vi "Calc_Remaining_Time.vi"(0 "Table In":T1[](array[typedef]) {"Carrier_2 Q (l/min)" format="%#.2f"; "Row Duration (mins)" format="%#.1f"; "Row No" min=0; "Trace Gas Concentration (%)" min=0.0 format="%#_4f"; "Carrier_1 Q (l/min)" format="%#.4f"; "Start X" format="%#.2f"; "Start Y" format="%#.2f"; "Start Z" format="%#.2f"; "End X" format="%#.2f"; "End Y" format="%#.2f"; "End Z" format="%#.2f"; "Tunnel Speed" format="%#.2f"; "Averaging time (mins)" min=0.0 format="%#.2f"}, 1 "Currently on Row":i32) -> (2 "Table Out":T1[](array[typedef]) {"Carrier_2 Q (l/min)" format="%#.2f"; "Row Duration (mins)" format="%#.1f"; "Row No" min=0; "Trace Gas Concentration (%)" min=0.0 format="%#_4f"; "Carrier_1 Q (l/min)" format="%#.4f"; "Start X" format="%#.2f"; "Start Y" format="%#.2f"; "Start Z" format="%#.2f"; "End X" format="%#.2f"; "End Y" format="%#.2f"; "End Z" format="%#.2f"; "Tunnel Speed" format="%#.2f"; "Averaging time (mins)" min=0.0 format="%#.2f"}, 3 "Estimated Completion time":string, 4 "noWaitCompletion":timestamp format="%<%H:%M\n%a %d>T", 5 "remainingTime":string)   [LabVIEW 2020]
uses:
  Traverse_cluster.ctl
  Spacing.ctl
  Controls/Multi_run_mode.ctl
  Controls/Overhead.ctl
  Globals/Extra_Commands_Global.vi
  Globals/Trav_pos_global.vi
panel:
  # "X           Y          Z"
  # "Start"
  # "End"
  # "X           Y          Z"
  # "Start"
  # "End"
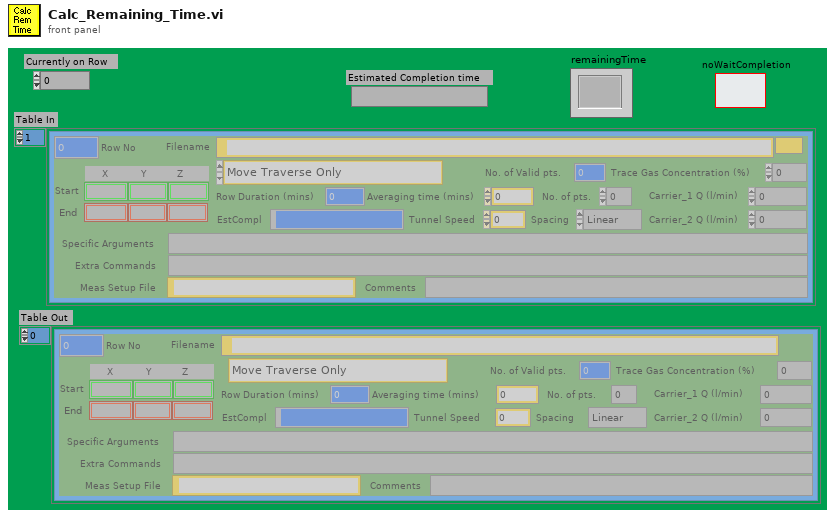
[diagram p1: front panel]
types:
  T1 = typedef "Traverse_cluster.ctl" = cluster{"Start X":sgl, "Start Y":sgl, "Start Z":sgl, "End X":sgl, "End Y":sgl, "End Z":sgl, "No. of pts.":i32, "Spacing":T2, "Filename":path, "Tunnel Speed":dbl, "Averaging time (mins)":dbl, "Extra Commands":string, "Carrier_1 Q (l/min)":dbl, "Carrier_2 Q (l/min)":dbl, "Trace Gas Concentration (%)":dbl, "Specific Arguments":string, "Comments":string, "Row No":i32, "Row Type Selector":T3, "EstCompl":string, "Row Duration (mins)":dbl, "No. of Valid pts.":i32, "Meas Setup File":string}
  T2 = typedef "Spacing.ctl" = enum16{"Linear", "Log", "Gauss", "Specified", "N/A"}
  T3 = typedef "Multi_run_mode.ctl" = enum16{"Move Traverse Only", "Set Tunnel Speed Only", "Set Source Only", "Set Measurement Conditions", "Single Measurement", "Vertical Profile", "Lateral Profile", "Longitudinal Profile", "Multi-Axis Profile", "Explore Volume", "Auto Calibrate", "Meas Fast FID Bkgnd", "Check Beam Power", "Scanning Valve Measurement", "Run VI Named:", "Set ADAM Ch", "Wait (minutes)", "Send Message", "Synchronize With:", "Fall Back to this Row", "Turn Off Row Repeating", "Traverse 3D Volume", "Blank Row", "Jump to Fall Back Row"}
  T4 = typedef "Overhead.ctl" = enum16{"Update total times", "Read Current Overhead", "Re Scale totals to 3 hrs", "Initialise totals to 3hr"}
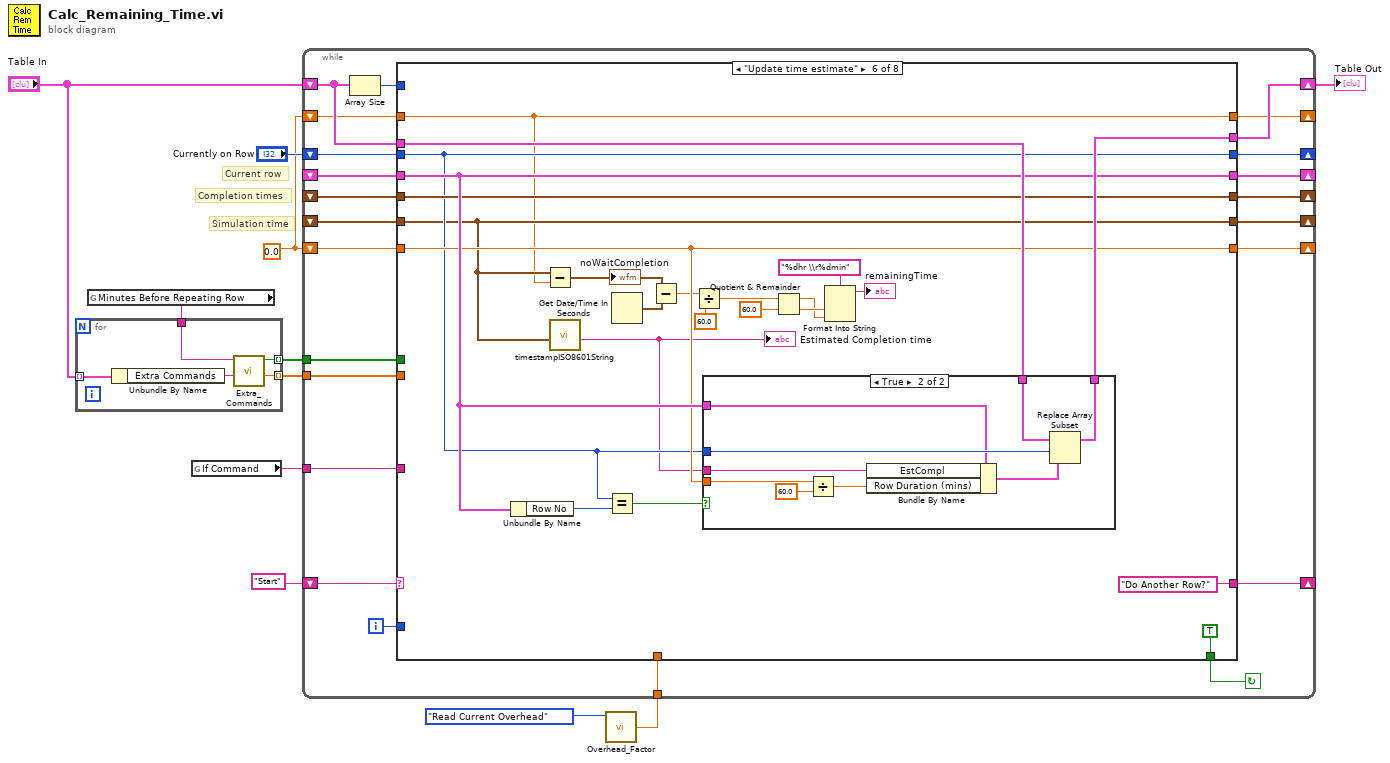
[diagram p0: block diagram]
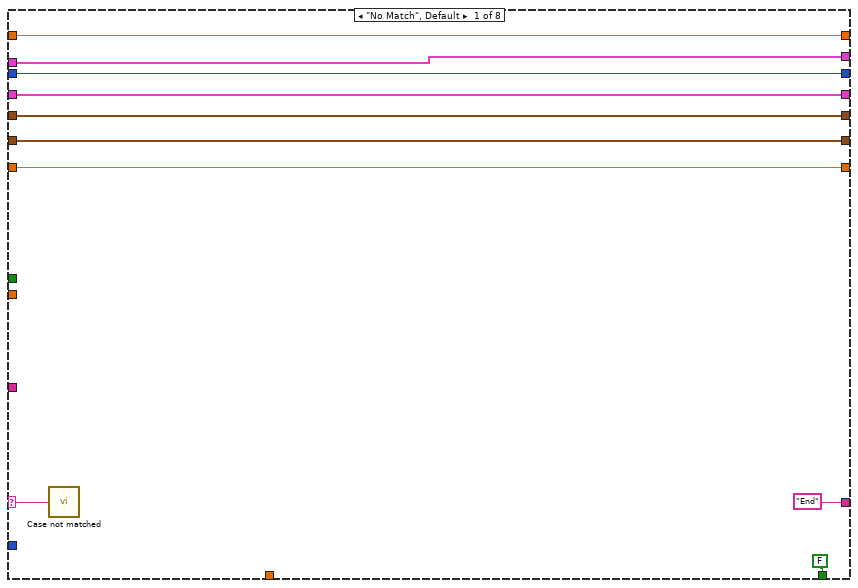
[diagram p2: hidden frame]
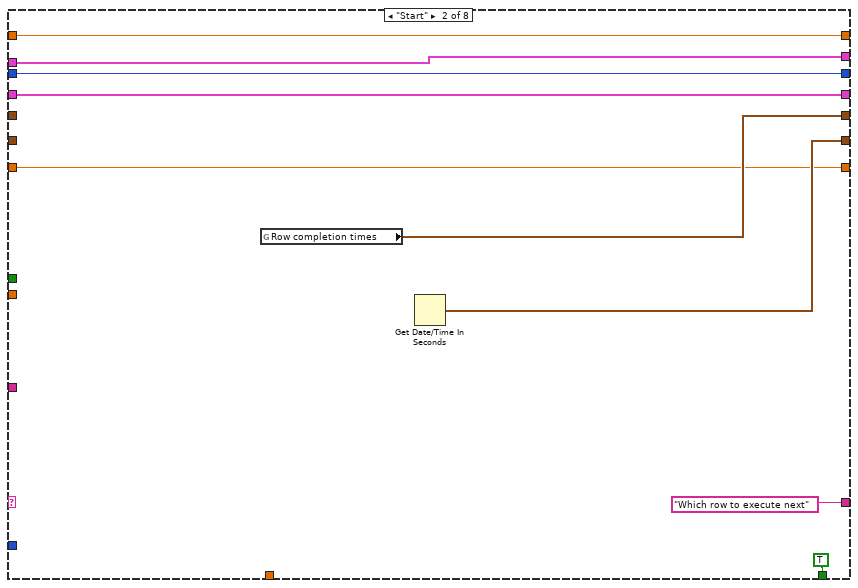
[diagram p3: hidden frame]
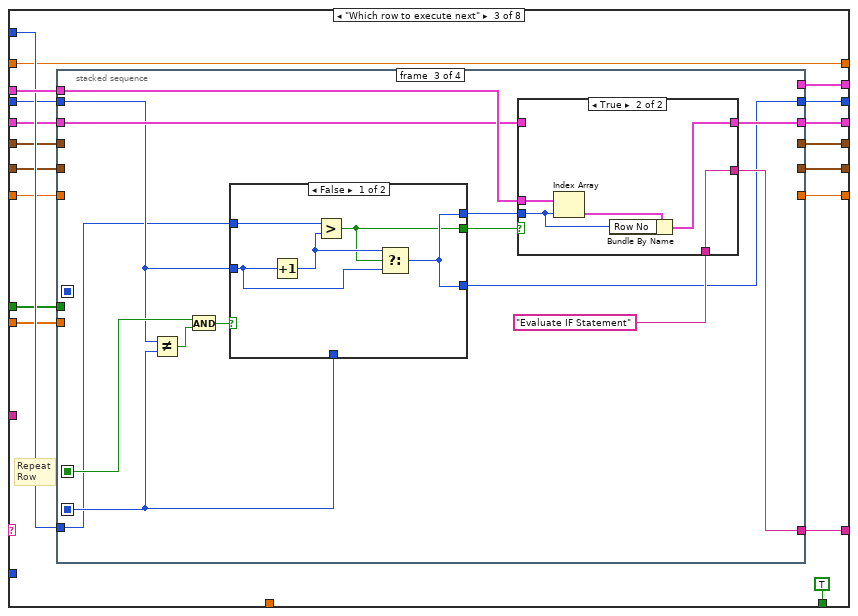
[diagram p4: hidden frame]
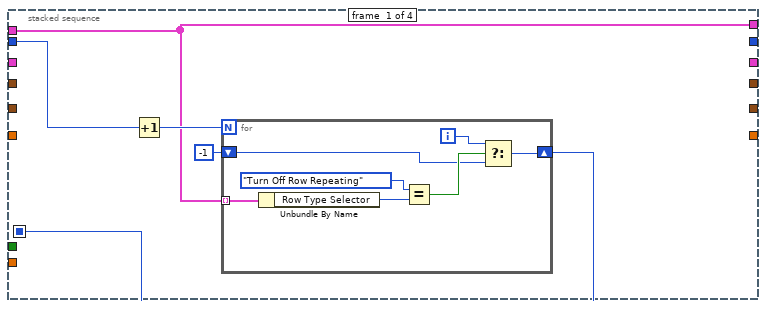
[diagram p5: hidden frame]
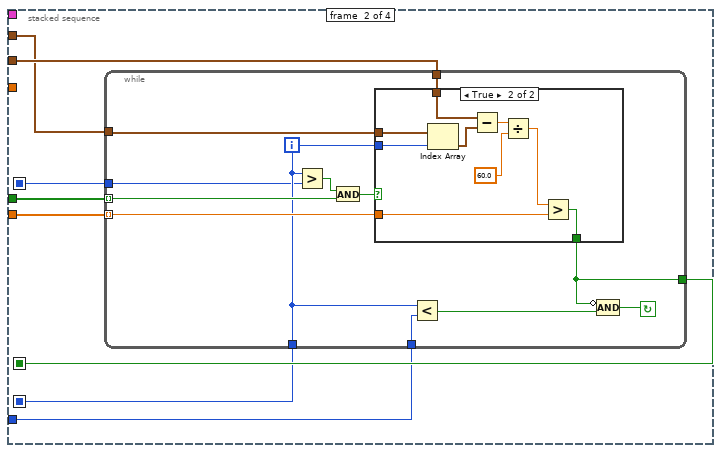
[diagram p6: hidden frame]
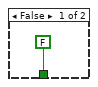
[diagram p7: hidden frame]
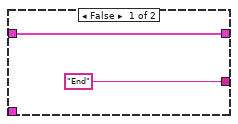
[diagram p8: hidden frame]
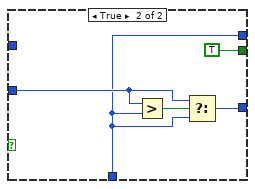
[diagram p9: hidden frame]
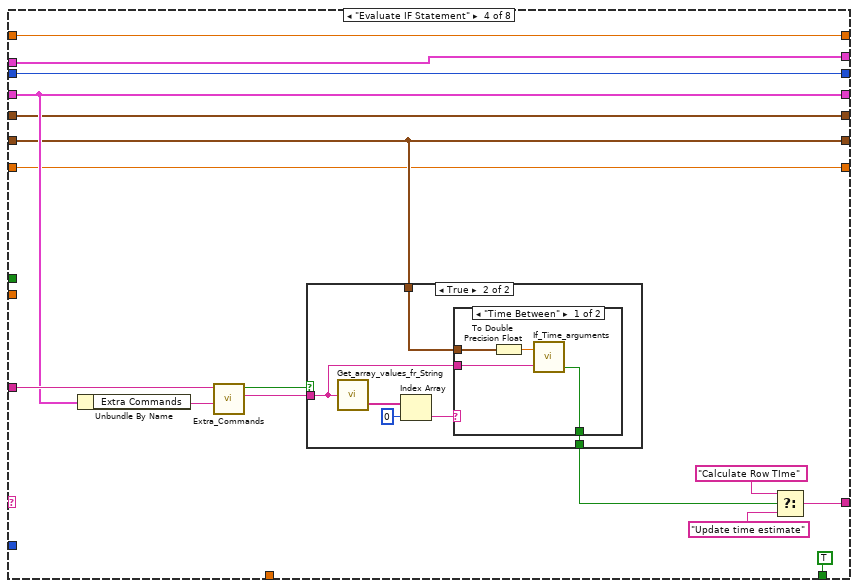
[diagram p11: hidden frame]
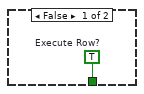
[diagram p12: hidden frame]
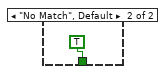
[diagram p13: hidden frame]
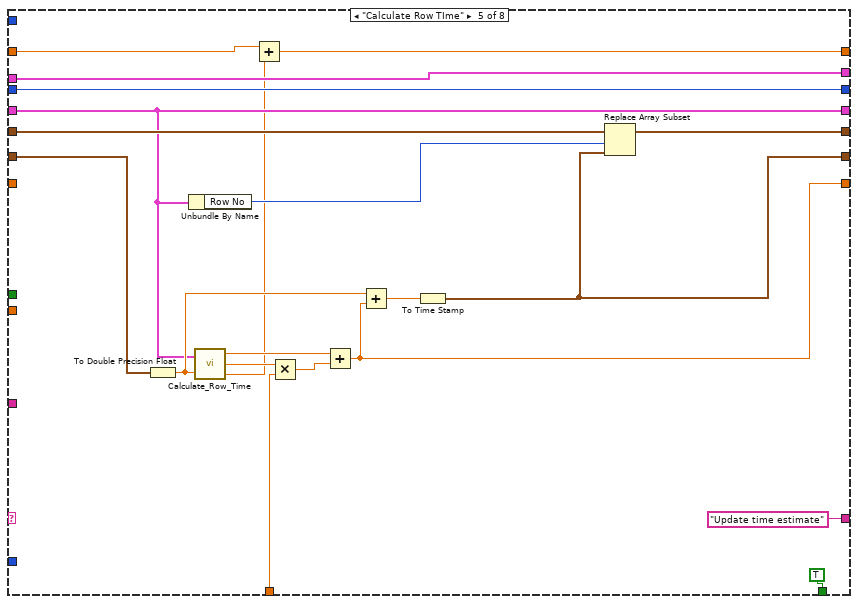
[diagram p14: hidden frame]
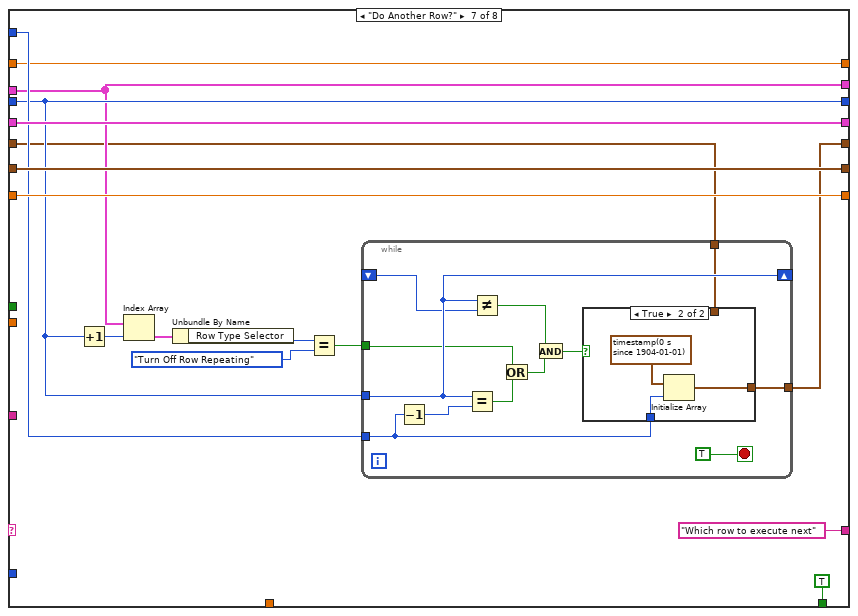
[diagram p16: hidden frame]
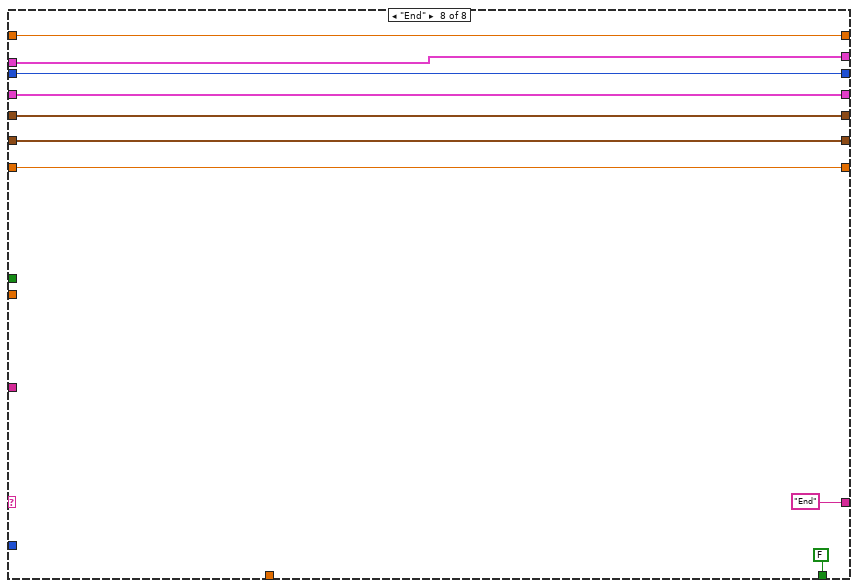
[diagram p18: hidden frame]
diagram:
  w1 = 0.0 ("row Duration")
  # "Simulation time"
  # "Completion times"
  # "Current row"
  n1 = global read "Extra_Commands_Global.vi" "Minutes Before Repeating Row"() -> (w2:string)
  n2 = for {
    tunnel: "Table In" -> [w15] mode=indexing
    tunnel: [w14] -> w4 mode=indexing
    tunnel: [w13] -> w3 mode=indexing
    tunnel: w2 -> [w12]
    n3 = Unbundle By Name(w15) -> ("Extra Commands"=w16:string)
    n4 = call "Extra_Commands.vi"("String to Search"=w16, "Command"=w12) -> ("Numeric Value"=w13:dbl, "Command Found"=w14:bool)  [unwired: 1 in, 3 out]
  }
  n5 = global read "Extra_Commands_Global.vi" "If Command"() -> (w7:string)
  n6 = call "Overhead_Factor.vi"("Mode"=Overhead."Read Current Overhead") -> ("Current Overhead Factor"=w8:dbl)  [unwired: 3 in]
  n7 = while {
    shift-left: "Start" -> [w37]
    shift-right: [w36] -> _
    shift-right: [w34] -> w10
    shift-left: "Table In" -> [w23]
    tunnel: w8 -> [w33]
    shift-right: [w32] -> _
    shift-left: _ -> [w31]
    shift-right: [w27] -> _
    shift-left: _ -> [w28]
    shift-right: [w29] -> _
    shift-left: _ -> [w30]
    shift-right: [w24] -> _
    shift-left: "Currently on Row" -> [w25]
    tunnel: w7 -> [w26]
    shift-right: [w22] -> _
    shift-left: w1 -> [w21]
    tunnel: w4 -> [w20]
    tunnel: w3 -> [w19]
    shift-right: [w17] -> _
    shift-left: w1 -> [w18]
    i -> [w38]
    stop <- w39 continue-if-true
    n8 = Array Size(array=w23) -> (size(s)=w35:i32)
    n9 = case shown="\"Update time estimate\"" w37 {
      selector: w37 -> [w41 _ _ _ _ _ _ _]
      tunnel: [FALSE ("Continue?") TRUE ("Continue?") TRUE ("Continue?") TRUE TRUE TRUE TRUE FALSE] -> w39
      tunnel: w23 -> [w49 w58 w74 w165 w199 w222 w237 w273]
      tunnel: w38 -> [_ _ _ _ _ _ _ _]
      tunnel: ["End" "Which row to execute next" w72 w167 "Update time estimate" "Do Another Row?" "Which row to execute next" "End"] -> w36
      tunnel: w35 -> [_ _ w73 _ _ _ w243 _]
      tunnel: [w49 w58 w75 w165 w199 w221 w237 w273] -> w34
      tunnel: w33 -> [_ _ _ _ w192 _ _ _]
      tunnel: [w46 w53 w71 w157 w186 w217 w247 w271] -> w32
      tunnel: w31 -> [w46 w53 w70 w157 w186 w217 w247 w271]
      tunnel: w30 -> [w43 _ w69 w155 w187 w212 w246 w269]
      tunnel: [w43 w55 w64 w155 w190 w212 w246 w269] -> w29
      tunnel: w28 -> [w44 _ w68 w156 w189 w216 w235 w270]
      tunnel: [w44 w54 w65 w156 w188 w216 w244 w270] -> w27
      tunnel: w26 -> [_ _ _ w159 _ _ _ _]
      tunnel: w25 -> [w45 w52 w67 w158 w185 w214 w238 w268]
      tunnel: [w45 w52 w66 w158 w185 w214 w238 w268] -> w24
      tunnel: [w42 w51 w62 w154 w184 w215 w245 w267] -> w22
      tunnel: w21 -> [w42 w51 w63 w154 _ w215 w245 w267]
      tunnel: w20 -> [_ _ w61 _ _ _ _ _]
      tunnel: w19 -> [_ _ w60 _ _ _ _ _]
      tunnel: w18 -> [w40 w50 w59 w153 w182 w211 w234 w266]
      tunnel: [w40 w50 w59 w153 w181 w211 w234 w266] -> w17
      frame "No Match", Default {
        n10 = call "Case not matched.vi"("Case Name not Matched"=w41) -> ()
      }
      frame "Start" {
        n11 = global read "Trav_pos_global.vi" "Row completion times"() -> (w54:timestamp[])
        n12 = Get Date/Time In Seconds() -> (seconds since 1Jan1904=w55:timestamp)
      }
      frame "Which row to execute next" {
        # "Repeat\nRow"
        n13 = stacked-sequence {
          seq-local: [_ w96 _ _] -> [_ _ w127 _]
          seq-local: [_ w95 _ _] -> [_ _ w128 _]
          seq-local: [w77 _ _ _] -> [_ w94 _ _]
          tunnel: [w78 _ _ _] -> w75
          tunnel: w74 -> [w78 _ w131 _]
          tunnel: w73 -> [_ w91 w120 _]
          tunnel: [_ _ w129 _] -> w72
          tunnel: [_ _ w123 _] -> w71
          tunnel: w70 -> [_ _ w122 _]
          tunnel: w69 -> [_ w93 _ w151]
          tunnel: w68 -> [_ w92 _ w152]
          tunnel: w67 -> [w81 _ w121 _]
          tunnel: [_ _ w119 _] -> w66
          tunnel: [_ _ _ w152] -> w65
          tunnel: [_ _ _ w151] -> w64
          tunnel: w63 -> [_ _ _ w150]
          tunnel: [_ _ _ w150] -> w62
          tunnel: w61 -> [_ w90 _ _]
          tunnel: w60 -> [_ w89 _ _]
          frame #0 {
            n14 = Increment(x=w81) -> (x+1=w79:i32)
            n15 = for {
              N: w79 -> [_]
              tunnel: w78 -> [w88] mode=indexing
              shift-right: [w85] -> w77
              shift-left: -1 -> [w82]
              i -> [w83]
              n16 = Unbundle By Name(w88) -> ("Row Type Selector"=w87:T3)
              n17 = Equal?(x=Multi_run_mode."Turn Off Row Repeating" ("Row Type Selector"), y=w87) -> (x = y?=w84:bool)
              n18 = Select(t=w83, s=w84, f=w82) -> (s? t:f=w85:i32)
            }
          }
          frame #1 {
            n19 = while {
              tunnel: w92 -> [w108]
              tunnel: w93 -> [w107]
              tunnel: [w102] -> w96
              tunnel: [w99] -> w95
              tunnel: w94 -> [w98]
              tunnel: w91 -> [w103]
              tunnel: w90 -> [w101] mode=indexing
              tunnel: w89 -> [w100] mode=indexing
              i -> [w99]
              stop <- w106 continue-if-true
              n20 = Greater?(x=w99, y=w98) -> (0:w97:bool)
              n21 = And(x=w97, y=w101) -> (x .and. y?=w104:bool)
              n22 = case shown="True" w104 {
                tunnel: w108 -> [_ w114]
                tunnel: w107 -> [_ w115]
                tunnel: w99 -> [_ w113]
                tunnel: w100 -> [_ w111]
                tunnel: [FALSE w110] -> w102
                frame False {
                }
                frame True {
                  n23 = Index Array(array=w114, index=w113) -> (element=w116:timestamp)
                  n24 = Subtract(x=w115, y=w116) -> (x-y=w117:dbl)
                  n25 = Divide(x=w117, y=60.0) -> (x/y=w112:dbl)
                  n26 = Greater?(x=w112, y=w111) -> (0:w110:bool)
                }
              }
              n27 = Less?(x=w99, y=w103) -> (x < y?=w105:bool)
              n28 = Compound Arithmetic op=AND(invert w102, w105) -> (w106:bool)
            }
          }
          frame #2 {
            n29 = Not Equal?(x=w121, y=w128) -> (x != y?=w126:bool)
            n30 = And(x=w127, y=w126) -> (x .and. y?=w125:bool)
            n31 = case shown="False" w125 {
              tunnel: w128 -> [_ w146]
              tunnel: w121 -> [w142 w148]
              tunnel: [w141 w147] -> w119
              tunnel: [w141 w146] -> w132
              tunnel: w120 -> [w144 _]
              tunnel: [w140 TRUE] -> w130
              frame False {
                n32 = Increment(x=w142) -> (x+1=w143:i32)
                n33 = Greater?(x=w144, y=w143) -> (0:w140:bool)
                n34 = Select(t=w143, s=w140, f=w142) -> (s? t:f=w141:i32)
              }
              frame True {
                n35 = Greater?(x=w148, y=w146) -> (0:w149:bool)
                n36 = Select(t=w148, s=w149, f=w146) -> (s? t:f=w147:i32)
              }
            }
            n37 = case shown="True" w130 {
              tunnel: w132 -> [_ w136]
              tunnel: w131 -> [_ w139]
              tunnel: ["End" w138] -> w129
              tunnel: "Evaluate IF Statement" -> [_ w138]
              tunnel: [w133 w135] -> w123
              tunnel: w122 -> [w133 _]
              frame False {
              }
              frame True {
                n38 = Index Array(array=w139, index=w136) -> (element=w137:T1)
                n39 = Bundle By Name(cluster=w137, "Row No"=w136) -> (w135:T1)
              }
            }
          }
          frame #3 {
          }
        }
      }
      frame "Evaluate IF Statement" {
        n40 = Unbundle By Name(w157) -> ("Extra Commands"=w164:string)
        n41 = call "Extra_Commands.vi"("String to Search"=w164, "Command"=w159) -> ("String Value"=w166:string, "Command Found"=w162:bool)  [unwired: 1 in, 3 out]
        n42 = case shown="True" w162 {
          tunnel: w166 -> [_ w172]
          tunnel: [w169 w171] -> w163
          tunnel: w155 -> [_ w170]
          frame False {
            w169 = TRUE  # Execute Row?
          }
          frame True {
            n43 = call "Get_array_values_fr_String.vi"("String Value"=w172) -> ("String array"=w174:string[])  [unwired: 1 out]
            n44 = Index Array(array=w174, index=0 ("Index")) -> (element=w173:string)
            n45 = case shown="\"Time Between\"" w173 {
              tunnel: w172 -> [w179 _]
              tunnel: [w178 TRUE ("Execute Row?")] -> w171
              tunnel: w170 -> [w176 _]
              frame "Time Between" {
                n46 = To Double Precision Float(number=w176) -> (double precision float=w177:dbl)
                n47 = call "If_Time_arguments.vi"("seconds since 1Jan1904"=w177, "String Value"=w179) -> ("Execute Row?"=w178:bool)  [unwired: 2 out]
              }
              frame "No Match", Default {
              }
            }
          }
        }
        n48 = Select(t="Calculate Row TIme", s=w163, f="Update time estimate") -> (s? t:f=w167:string)
      }
      frame "Calculate Row TIme" {
        n49 = To Double Precision Float(number=w187) -> (double precision float=w195:dbl)
        n50 = Unbundle By Name(w186) -> ("Row No"=w198:i32)
        n51 = call "Calculate_Row_Time.vi"("Multi Run Row"=w186, "Row Start Time (Sec Since 1904)"=w195) -> ("Fixed Time (Sec)"=w196:dbl, "Scalable Time (Sec)"=w193:dbl, "waitTime (Sec)"=w183:dbl)
        n52 = Add(x=w182, y=w183) -> (x+y=w181:dbl)
        n53 = Multiply(x=w193, y=w192) -> (x*y=w197:dbl)
        n54 = Add(x=w196, y=w197) -> (x+y=w184:dbl)
        n55 = Add(x=w195, y=w184) -> (x+y=w194:dbl)
        n56 = To Time Stamp(1:w194) -> (0:w190:timestamp)
        n57 = Replace Array Subset(array=w189, new element=w190, index=w198) -> (w188:timestamp[])
      }
      frame "Update time estimate" {
        n58 = Unbundle By Name(w217) -> ("Row No"=w220:i32)
        n59 = Subtract(x=w212, y=w211) -> (x-y=w210:timestamp)
        "noWaitCompletion" <- w210
        n60 = call "timestampISO8601String.vi"("Time Stamp"=w212) -> ("date/time"=w213:string)  [unwired: 7 in, 3 out]
        "Estimated Completion time" <- w213
        n61 = Equal?(x=w214, y=w220) -> (x = y?=w219:bool)
        n62 = Get Date/Time In Seconds() -> (seconds since 1Jan1904=w209:timestamp)
        n63 = Subtract(x=w210, y=w209) -> (x-y=w208:dbl)
        n64 = Divide(x=w208, y=60.0) -> (x/y=w206:dbl)
        n65 = case shown="True" w219 {
          tunnel: w214 -> [_ w233]
          tunnel: w222 -> [w224 w232]
          tunnel: [w224 w230] -> w221
          tunnel: w213 -> [_ w229]
          tunnel: w217 -> [_ w228]
          tunnel: w215 -> [_ w225]
          frame False {
          }
          frame True {
            n66 = Divide(x=w225, y=60.0) -> (x/y=w226:dbl)
            n67 = Bundle By Name(cluster=w228, "EstCompl"=w229, "Row Duration (mins)"=w226) -> (w231:T1)
            n68 = Replace Array Subset(array=w232, new element=w231, index=w233) -> (w230:T1[])
          }
        }
        n69 = Quotient & Remainder(x=w206, y=60.0) -> (x-y*floor(x/y)=w203:dbl, floor(x/y)=w204:dbl)
        n70 = Format Into String(format string="%dhr \\r%dmin", w204, w203) -> (resulting string=→"remainingTime":string)  [unwired: 2 in, 1 out]
      }
      frame "Do Another Row?" {
        n71 = Increment(x=w238) -> (x+1=w241:i32)
        n72 = Index Array(array=w237, index=w241) -> (element=w242:T1)
        n73 = Unbundle By Name(w242) -> ("Row Type Selector"=w239:T3)
        n74 = Equal?(x=w239, y=Multi_run_mode."Turn Off Row Repeating" ("Row Type Selector")) -> (x = y?=w236:bool)
        n75 = while {
          shift-right: [w260] -> _
          shift-left: _ -> [w259]
          tunnel: w243 -> [w256]
          tunnel: w238 -> [w260]
          tunnel: w236 -> [w253]
          tunnel: [w251] -> w244
          tunnel: w235 -> [w250]
          stop <- TRUE stop-if-true
          n76 = Decrement(x=w256) -> (x-1=w261:i32)
          n77 = Equal?(x=w260, y=w261) -> (x = y?=w254:bool)
          n78 = Not Equal?(x=w260, y=w259) -> (x != y?=w258:bool)
          n79 = Or(x=w253, y=w254) -> (x .or. y?=w252:bool)
          n80 = And(x=w258, y=w252) -> (x .and. y?=w257:bool)
          n81 = case shown="True" w257 {
            tunnel: w256 -> [_ w264]
            tunnel: [w262 w263] -> w251
            tunnel: w250 -> [w262 _]
            frame False {
            }
            frame True {
              n82 = Initialize Array(timestamp(0 s since 1904-01-01) ("seconds since 1Jan1904"), w264) -> (w263:timestamp[])
            }
          }
        }
      }
      frame "End" {
      }
    }
  }
  "Table Out" <- w10
